vi "CSM - Post Message.vi"(7 "Current Module(\"\" to generate a ID)":string, 8 "Error In (no error)":errorcluster, 9 "Target Module":string="Target", 10 "Arguments (\"\")":string, 11 "State":string="API State") -> (0 "error out":errorcluster)   [LabVIEW 2020, in "Communicable State Machine.lvlib"]
doc: "Post a message to CSM specified.\n\n<b>Inputs:</b>\n - <b>Target Module</b>:Target CSM Module name.\n - <b>State</b>: Message to post.\n - <b>Arguments (\"\")</b>: Argument of the message.\n - <b>Error In (no error)</b>: Error cluster\n\n<b>Outputs:</b>\n - <b>error out</b>: Error cluster"
uses:
  Communicable State Machine.lvlib
  _CSM_MSG_TYPE.ctl
  Priority Queue.lvclass/Priority Queue.ctl
  _CSMObj-Message Check.vi
  _CSMObj-Enqueue Cross-Module Message.vi
  _CSMOFGV Get.vi
  Enqueue Element.vi
  _CSMOFGV.vi
  CSM Not Allowed Message.vi
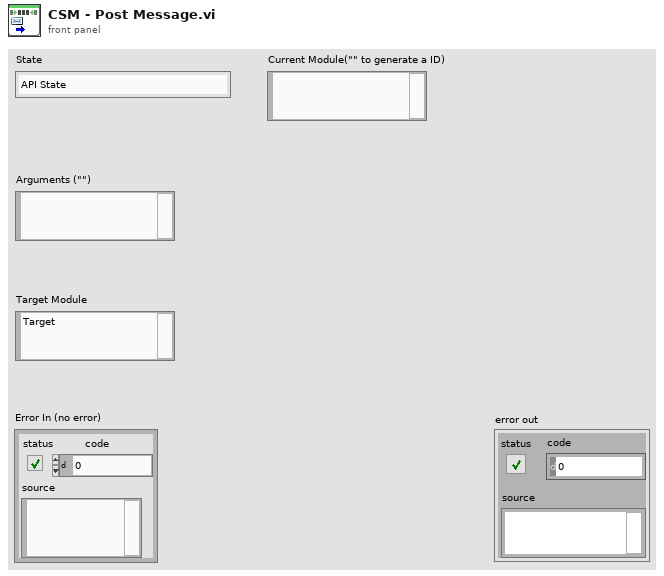
[diagram p1: front panel]
types:
  T1 = typedef "Communicable State Machine.lvlib/_CSM_MSG_TYPE.ctl" = enum16{"Sync Message(-@)", "Async Message(->)", "Async without Response(->|)", "Async Response", "Broadcast(-><all>)", "Broadcast(-><status>)", "Broadcast(-><interrupt>)", "Append to JKISM States", "Append to JKISM States(High Priority)"}
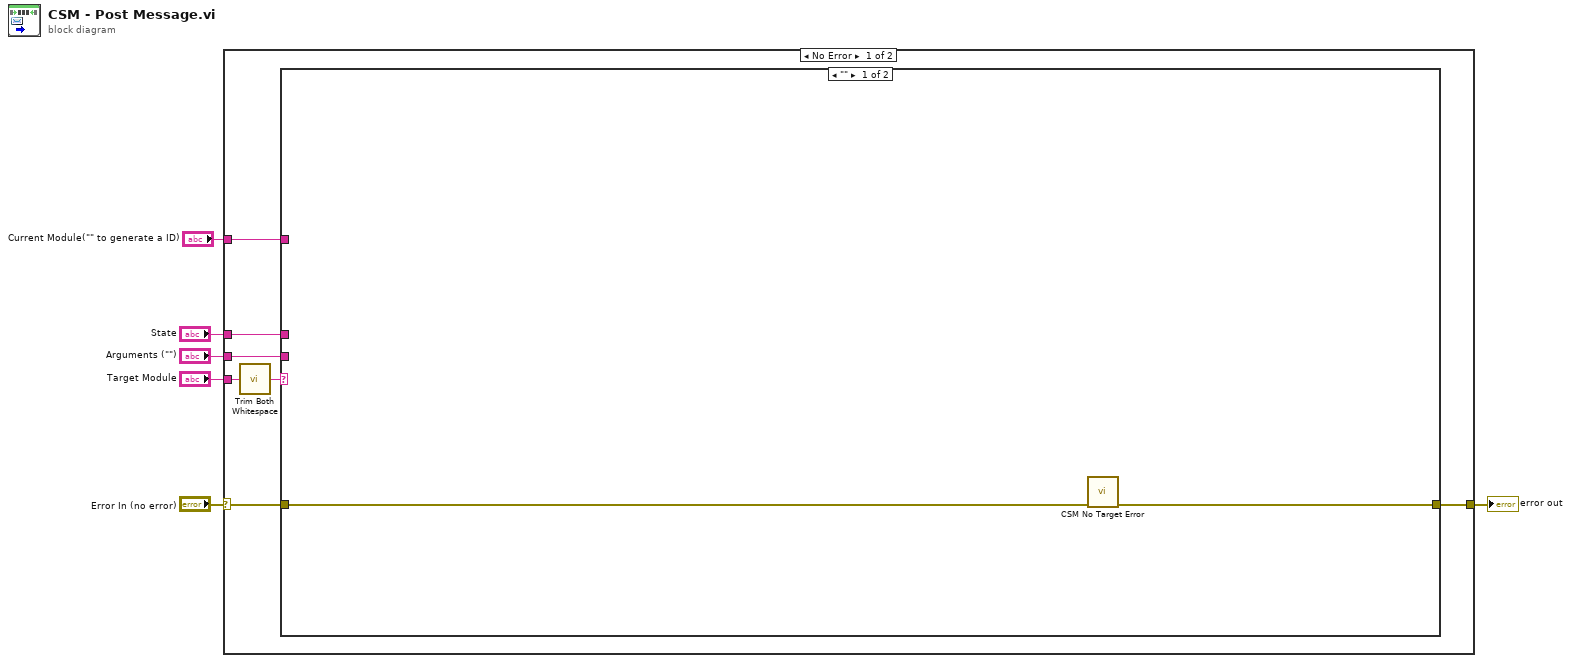
[diagram p0: block diagram]
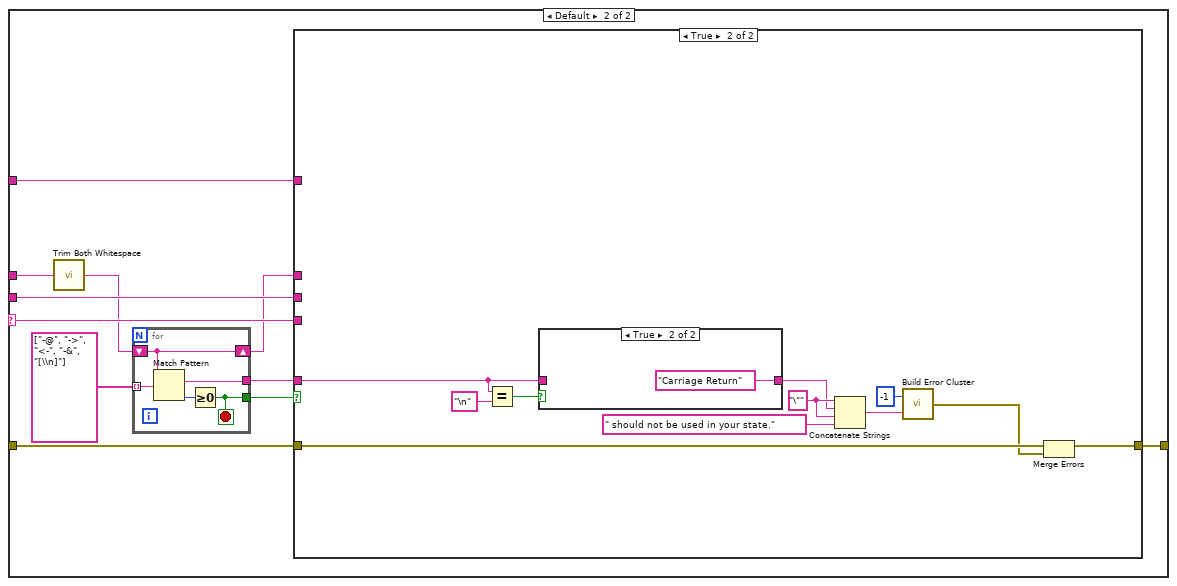
[diagram p2: hidden frame]
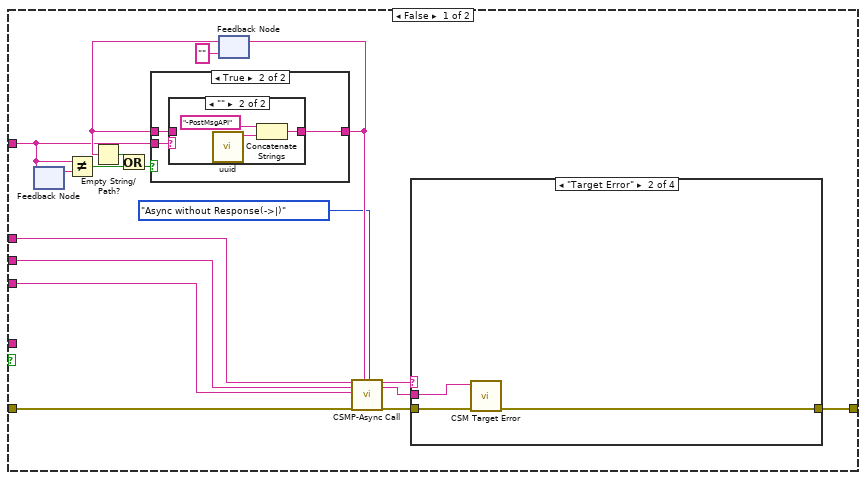
[diagram p3: hidden frame]
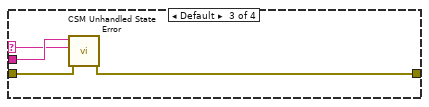
[diagram p7: hidden frame]
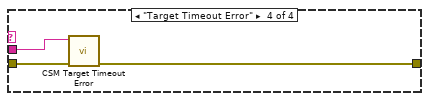
[diagram p8: hidden frame]
diagram:
  n1 = case shown="No Error" "Error In (no error)" {
    selector: "Error In (no error)" -> [w11 w81]
    tunnel: "State" -> [w8 _]
    tunnel: [w12 w81] -> w4
    tunnel: "Arguments (\"\")" -> [w9 _]
    tunnel: "Target Module" -> [w13 _]
    tunnel: "Current Module(\"\" to generate a ID)" -> [w7 _]
    frame No Error {
      n2 = call "Trim Both Whitespace.vi"("string"=w13) -> ("trimmed string"=w10:string)  [unwired: 1 in]
      n3 = case shown="\"\"" w10 {
        selector: w10 -> [_ w25]
        tunnel: w8 -> [_ w21]
        tunnel: w9 -> [_ w26]
        tunnel: [w14 w24] -> w12
        tunnel: w11 -> [w15 w23]
        tunnel: w7 -> [_ w16]
        frame "" {
          n4 = call "CSM No Target Error.vi"("error in (no error)"=w15) -> ("error out"=w14:errorcluster)  [unwired: 10 in]
        }
        frame Default {
          n5 = call "Trim Both Whitespace.vi"("string"=w21) -> ("trimmed string"=w17:string)  [unwired: 1 in]
          n6 = for {
            shift-right: [w80] -> w20
            shift-left: w17 -> [w80]
            tunnel: string[] ["-@", "->", "<-", "-&", "[\\n]"] -> [w79] mode=indexing
            tunnel: [w77] -> w18
            tunnel: [w76] -> w19
            stop <- w76 stop-if-true
            n7 = Match Pattern(string=w80, regular expression=w79) -> (match substring=w77:string, offset past match=w78:i32)  [unwired: 1 in, 2 out]
            n8 = Greater Or Equal To 0?(x=w78) -> (x >= 0?=w76:bool)
          }
          n9 = case shown="True" w19 {
            tunnel: w26 -> [w29 _]
            tunnel: w25 -> [w28 _]
            tunnel: [w27 w65] -> w24
            tunnel: w23 -> [w33 w66]
            tunnel: w20 -> [w31 _]
            tunnel: w18 -> [_ w63]
            tunnel: w16 -> [w32 _]
            frame False {
              n10 = feedback #1() -> (w39:string)  [unwired: 1 in]
              n11 = feedback-in #1(w32) -> ()
              n12 = Not Equal?(x=w32, y=w39) -> (x != y?=w38:bool)
              n13 = feedback #2("") -> (w35:string)
              n14 = Empty String/Path?(string/path=w35) -> (empty?=w34:bool)
              n15 = Or(x=w34, y=w38) -> (x .or. y?=w36:bool)
              n16 = case shown="True" w36 {
                tunnel: w35 -> [w44 w47]
                tunnel: w32 -> [_ w46]
                tunnel: [w44 w45] -> w40
                frame False {
                }
                frame True {
                  n17 = case shown="\"\"" w46 {
                    selector: w46 -> [w48 _]
                    tunnel: [w48 w49] -> w45
                    tunnel: w47 -> [_ _]
                    frame Default {
                    }
                    frame "" {
                      n18 = call "uuid.vi"() -> ("UUID"=w50:string)  [unwired: 11 in]
                      n19 = Concatenate Strings("-PostMsgAPI" ("Name(\"\" to use uuid)"), w50) -> (w49:string)
                    }
                  }
                }
              }
              n20 = feedback-in #2(w40) -> ()
              n21 = call "CSMP-Async Call.vi"("state"=w31, "args"=w29, "source/target"=w28, "Error in"=w33, "Module Name"=w40, "Msg Type"=_CSM_MSG_TYPE."Async without Response(->|)") -> ("state out"=w43:string, "args out"=w41:string, "error"=w42:errorcluster)  [unwired: 8 in, 3 out]
              n22 = case shown="\"Target Error\"" w43 {
                selector: w43 -> [_ _ w56 _]
                tunnel: w42 -> [w52 w54 w58 w61]
                tunnel: [w52 w53 w57 w60] -> w27
                tunnel: w41 -> [_ w55 w59 w62]
                frame "Async Message Posted" {
                }
                frame "Target Error" {
                  n23 = call "CSM Target Error.vi"("error in (no error)"=w54, "Arguments(as CSM Name)"=w55) -> ("error out"=w53:errorcluster)  [unwired: 9 in]
                }
                frame Default {
                  n24 = call "CSM Unhandled State Error.vi"("error in (no error)"=w58, "Current State"=w56, "CSM Name"=w59) -> ("error out"=w57:errorcluster)  [unwired: 8 in]
                }
                frame "Target Timeout Error" {
                  n25 = call "CSM Target Timeout Error.vi"("error in (no error)"=w61, "Arguments(as CSM Name)"=w62) -> ("error out"=w60:errorcluster)  [unwired: 9 in]
                }
              }
            }
            frame True {
              w70 = "\"" ("string")
              n26 = Equal?(x=w63, y="\n" ("regular expression")) -> (x = y?=w67:bool)
              n27 = case shown="True" w67 {
                tunnel: [w74 "Carriage Return" ("State")] -> w69
                tunnel: w63 -> [w74 _]
                frame False {
                }
                frame True {
                }
              }
              n28 = Concatenate Strings(w70, w69, w70, " should not be used in your state." ("String to Prepend to source (\"\")")) -> (w71:string)
              n29 = call "Build Error Cluster.vi"("String to Prepend to source (\"\")"=w71, "code"=-1) -> ("error out"=w64:errorcluster)
              n30 = Merge Errors(w66, w64) -> (w65:errorcluster)
            }
          }
        }
      }
    }
    frame Error {
    }
  }
  "error out" <- w4
